vi "USB2XXX_LINEX_MasterTest.vi"() -> ()   [LabVIEW 2010]
panel:
  in  "stop":bool
  in  "pInMsg 3":T1={"Timestamp"=20, "MsgType"=2, "CheckType"=1, "DataLen"=8, "Sync"=85, "PID"=3, "Data[0]"=33, "Data[1]"=34, "Data[2]"=35, "Data[3]"=36, "Data[4]"=37, "Data[5]"=38, "Data[6]"=39, "Data[7]"=40, "Check"=0, "Reserve"=0, "Reserve"=0} {"Sync" format="%x"; "PID" format="%x"; "Data[0]" format="%x"; "Data[1]" format="%x"; "Data[2]" format="%x"; "Data[3]" format="%x"; "Data[4]" format="%x"; "Data[5]" format="%x"; "Data[6]" format="%x"; "Data[7]" format="%x"; "Check" format="%x"; "Reserve" format="%x"; "Reserve" format="%x"}
  in  "pInMsg 2":T1={"Timestamp"=20, "MsgType"=2, "CheckType"=1, "DataLen"=8, "Sync"=85, "PID"=2, "Data[0]"=17, "Data[1]"=18, "Data[2]"=19, "Data[3]"=20, "Data[4]"=21, "Data[5]"=22, "Data[6]"=23, "Data[7]"=24, "Check"=0, "Reserve"=0, "Reserve"=0} {"Sync" format="%x"; "PID" format="%x"; "Data[0]" format="%x"; "Data[1]" format="%x"; "Data[2]" format="%x"; "Data[3]" format="%x"; "Data[4]" format="%x"; "Data[5]" format="%x"; "Data[6]" format="%x"; "Data[7]" format="%x"; "Check" format="%x"; "Reserve" format="%x"; "Reserve" format="%x"}
  out "pOutMsg":T2(array[cluster]) {"Sync" format="%x"; "PID" format="%x"; "Data[0]" format="%x"; "Data[1]" format="%x"; "Data[2]" format="%x"; "Data[3]" format="%x"; "Data[4]" format="%x"; "Data[5]" format="%x"; "Data[6]" format="%x"; "Data[7]" format="%x"; "Check" format="%x"}
  in  "pInMsg":T1={"Timestamp"=20, "MsgType"=1, "CheckType"=1, "DataLen"=8, "Sync"=85, "PID"=1, "Data[0]"=1, "Data[1]"=2, "Data[2]"=3, "Data[3]"=4, "Data[4]"=5, "Data[5]"=6, "Data[6]"=7, "Data[7]"=8, "Check"=0, "Reserve"=0, "Reserve"=0} {"Sync" format="%x"; "PID" format="%x"; "Data[0]" format="%x"; "Data[1]" format="%x"; "Data[2]" format="%x"; "Data[3]" format="%x"; "Data[4]" format="%x"; "Data[5]" format="%x"; "Data[6]" format="%x"; "Data[7]" format="%x"; "Check" format="%x"; "Reserve" format="%x"; "Reserve" format="%x"}
  out "function return":i32
  in  "BaudRate":u32=19200
  in  "Channel Index":u8(ring) items=["LIN1", "LIN2"]
  in  "Device Index":i32(ring) items=["0", "1", "2", "3", "4", "5"]
  # "波特率一定要设置，否则程序可能出错"
  # "同时发送3帧数据，第一帧为主机发送数据给从机，第二第三帧为主机向从机读取数据"
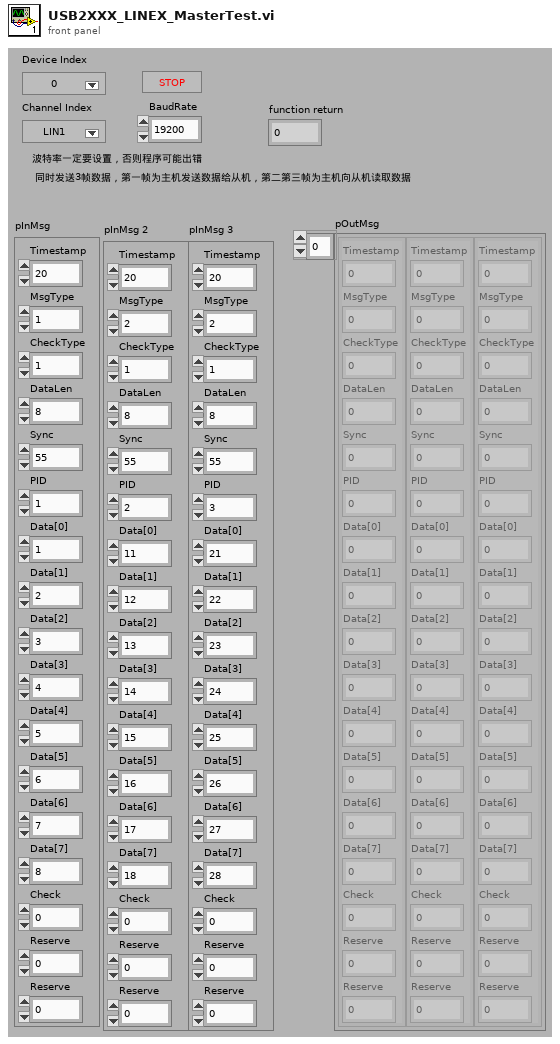
[diagram p1: front panel]
types:
  T1 = cluster{"Timestamp":u32, "MsgType":u8, "CheckType":u8, "DataLen":u8, "Sync":u8, "PID":u8, "Data[0]":u8, "Data[1]":u8, "Data[2]":u8, "Data[3]":u8, "Data[4]":u8, "Data[5]":u8, "Data[6]":u8, "Data[7]":u8, "Check":u8, "Reserve":u8, "Reserve":u8}
  T2 = cluster{"Timestamp":u32, "MsgType":u8, "CheckType":u8, "DataLen":u8, "Sync":u8, "PID":u8, "Data[0]":u8, "Data[1]":u8, "Data[2]":u8, "Data[3]":u8, "Data[4]":u8, "Data[5]":u8, "Data[6]":u8, "Data[7]":u8, "Check":u8, "Reserve":u8, "Reserve":u8}[]
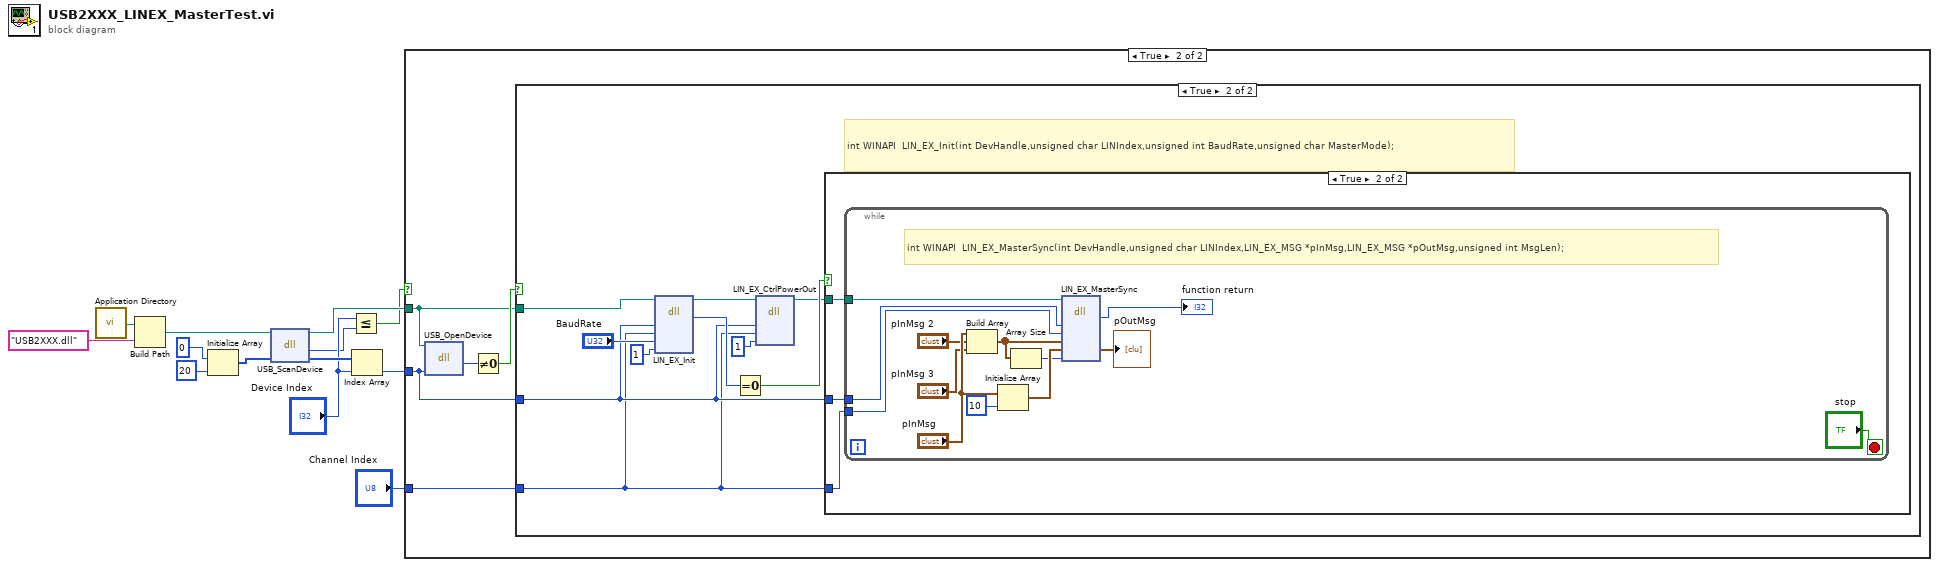
[diagram p0: block diagram]
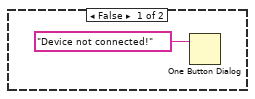
[diagram p2: hidden frame]
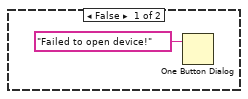
[diagram p3: hidden frame]
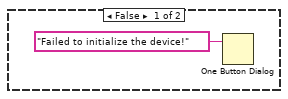
[diagram p4: hidden frame]
diagram:
  n1 = call <vilib>:"Application Directory.vi"() -> ("Application Directory"=w6:path)
  n2 = Build Path(base path=w6, name or relative path="USB2XXX.dll") -> (appended path=w5:path)
  n3 = Initialize Array(0, 20 ("dimension size")) -> (w10:i32[])
  n4 = dll-call lib="E:/OtherWork/STM32/USB2XXX_Example/examples/Labview/PublicFiles/USB2XXX.dll" fn="USB_ScanDevice"(path in=w5, "pDevNum"=w10) -> (path out=w8:path, "return type"=w2:i32, "pDevNum"=w13:i32[])  [unwired: 2 in, 1 out]
  n5 = Less Or Equal?(x="Device Index", y=w2) -> (x <= y?=w4:bool)
  n6 = Index Array(array=w13, index="Device Index") -> (element=w9:i32)
  n7 = case shown="True" w4 {
    tunnel: w9 -> [_ w17]
    tunnel: w8 -> [_ w16]
    tunnel: "Channel Index" -> [_ w15]
    frame False {
      n8 = One Button Dialog(message="Device not connected!") -> ()  [unwired: 1 in, 1 out]
    }
    frame True {
      n9 = dll-call lib="E:/OtherWork/STM32/USB2XXX_Example/examples/Labview/PublicFiles/USB2XXX.dll" fn="USB_OpenDevice"(path in=w16, "DevIndex"=w17) -> ("return type"=w19:u8)  [unwired: 3 in, 2 out]
      n10 = Not Equal To 0?(x=w19) -> (x != 0?=w18:bool)
      n11 = case shown="True" w18 {
        tunnel: w17 -> [_ w23]
        tunnel: w16 -> [_ w28]
        tunnel: w15 -> [_ w22]
        frame False {
          n12 = One Button Dialog(message="Failed to open device!") -> ()  [unwired: 1 in, 1 out]
        }
        frame True {
          # "int WINAPI  LIN_EX_Init(int DevHandle,unsigned char LINIndex,unsigned int BaudRate,unsigned char MasterMode);"
          n13 = dll-call lib="E:/OtherWork/STM32/USB2XXX_Example/examples/Labview/PublicFiles/USB2XXX.dll" fn="LIN_EX_Init"(path in=w28, "DevHandle"=w23, "LINIndex"=w22, "BaudRate"="BaudRate", "MasterMode"=u8 1) -> (path out=w25:path, "return type"=w27:i32)  [unwired: 6 in, 1 out]
          n14 = Equal To 0?(x=w27) -> (x = 0?=w26:bool)
          n15 = dll-call lib="E:/Projects/USB2XXX/trunk/USB2XXX/USB2XXX/vs2010/Release/USB2XXX.*" fn="LIN_EX_CtrlPowerOut"(path in=w25, "DevHandle"=w23, "LINIndex"=w22, "VbatValue"=u8 1 ("State")) -> (path out=w24:path)  [unwired: 6 in, 1 out]
          n16 = case shown="True" w26 {
            tunnel: w22 -> [_ w34]
            tunnel: w23 -> [_ w33]
            tunnel: w24 -> [_ w32]
            frame False {
              n17 = One Button Dialog(message="Failed to initialize the device!") -> ()  [unwired: 1 in, 1 out]
            }
            frame True {
              n18 = while {
                tunnel: w34 -> [w38]
                tunnel: w33 -> [w37]
                tunnel: w32 -> [w35]
                stop <- "stop" stop-if-true
                # "int WINAPI  LIN_EX_MasterSync(int DevHandle,unsigned char LINIndex,LIN_EX_MSG *pInMsg,LIN_EX_MSG *pOutMsg,unsigned int MsgLen);"
                n19 = Build Array("pInMsg", "pInMsg 2", "pInMsg 3") -> (w40:T2)
                n20 = Initialize Array("pInMsg", 10 ("dimension size")) -> (w41:T2)
                n21 = Array Size(array=w40) -> (size(s)=w39:i32)
                n22 = dll-call lib="E:/OtherWork/STM32/USB2XXX_Example/examples/Labview/PublicFiles/USB2XXX.dll" fn="LIN_EX_MasterSync"(path in=w35, "DevHandle"=w37, "LINIndex"=w38, "pInMsg"=w40, "pOutMsg"=w41, "MsgLen"=w39) -> ("return type"=→"function return":i32, "pOutMsg"=→"pOutMsg":T2)  [unwired: 6 in, 2 out]
              }
            }
          }
        }
      }
    }
  }
